vi "validate key value pair.vi"(8 "error in":errorcluster, 9 "value":string, 10 "key":string, 11 "BuckBoost configuration in":refnum<class "BuckBoost configuration.lvclass">) -> (0 "error out":errorcluster, 3 "BuckBoost configuration out":refnum<class "BuckBoost configuration.lvclass">)   [LabVIEW 2017, in "BuckBoost configuration.lvclass"]
uses:
  BuckBoost configuration.lvclass
  <vilib>/NI/DCAF/Tag Editor Core/control module/configuration/control module configuration.lvclass
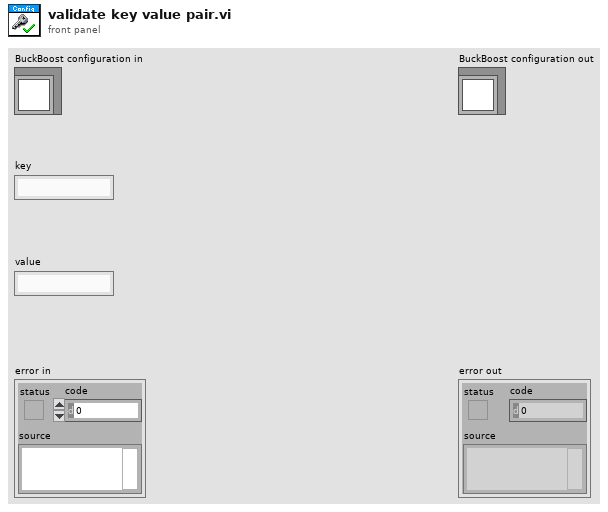
[diagram p1: front panel]
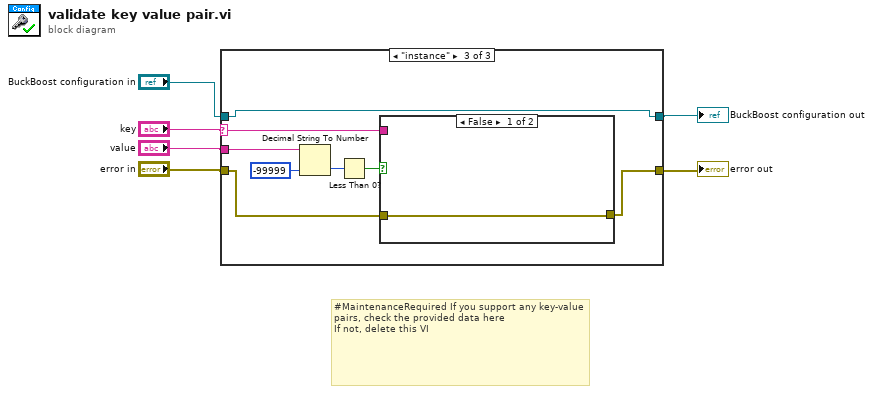
[diagram p0: block diagram]
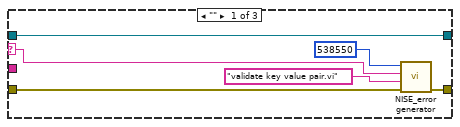
[diagram p2: hidden frame]
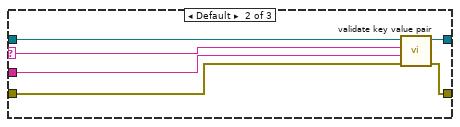
[diagram p3: hidden frame]
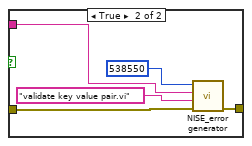
[diagram p4: hidden frame]
diagram:
  # "#MaintenanceRequired If you support any key-value pairs, check the provided data here\nIf not, delete this VI"
  n1 = case shown="\"instance\"" "key" {
    selector: "key" -> [w9 w13 w20]
    tunnel: [w7 w18 w21] -> w1
    tunnel: [w12 w17 w19] -> w6
    tunnel: "error in" -> [w8 w16 w23]
    tunnel: "value" -> [_ w15 w26]
    tunnel: "BuckBoost configuration in" -> [w12 w14 w19]
    frame "" {
      n2 = call <vilib>:"NISE_error generator.vi"("error in"=w8, "source"="validate key value pair.vi", "append error message"=w9, "error code (0)"=538550) -> ("error out"=w7:errorcluster)  [unwired: 5 in]
    }
    frame Default {
      n3 = call-parent "validate key value pair.vi"("error in"=w16, "value"=w15, "key"=w13, "fixed channel configuration in"=w14) -> ("error out"=w18:errorcluster, "fixed channel configuration out"=w17:refnum<class "BuckBoost configuration.lvclass">)  [unwired: 6 in]
    }
    frame "instance" {
      n4 = Decimal String To Number(string=w26, default (0L)=-99999 ("default (0 I32)")) -> (number=w24:i32)  [unwired: 1 in, 1 out]
      n5 = Less Than 0?(x=w24) -> (x < 0?=w22:bool)
      n6 = case shown="False" w22 {
        tunnel: w23 -> [w27 w30]
        tunnel: [w27 w29] -> w21
        tunnel: w20 -> [_ w28]
        frame False {
        }
        frame True {
          n7 = call <vilib>:"NISE_error generator.vi"("error in"=w30, "source"="validate key value pair.vi", "append error message"=w28, "error code (0)"=538550) -> ("error out"=w29:errorcluster)  [unwired: 5 in]
        }
      }
    }
  }
  "error out" <- w1
  "BuckBoost configuration out" <- w6
